vi "Config HW Extract.vi"(4 "Get(f) Set(t)":bool, 6 "Send Cmd Timout(ms)":u32=300, 7 "Drive Refs":T1={"DeviceStatus"={"status"=FALSE, "code"=0, "source"=""}, "Type"=enum."PWM", "PWM"={"PWM Channel"=enum."Invalid", "DeadBand"={"Name"="", "maxPositivePwm"=0, "minPositivePwm"=0, "centerPwm"=0, "maxNegativePwm"=0, "minNegativePwm"=0, "angularRange"=0}}, "CAN"={"Device Number"=0, "SetOutput VI Ref"=variant, "GetOutput VI Ref"=variant, "Enable VI Ref"=variant, "Disable VI Ref"=variant, "Data"=variant}, "Invert"=FALSE, "DIO PWM"={"PWM \"Enable\" Channel"=enum."Invalid", "DIOChannel"=enum."Invalid", "PWM Rate"=0.0}}, 8 "Error":errorcluster, 9 "HW Config":T6={"Drive"={"Drive HW Ver"=0, "SparkMax Output"={"Motor Invert"=FALSE, "Ramp Rate OL (S)"=1.0, "Dead Band"=0.0, "Idle Mode"=enum."Brake"}, "Slot 0 CL"={"Gains"={"P"=0.1, "I"=0.0, "D"=0.0, "F"=0.0}, "I Zone"=0.0, "Peak Out -1 0 1"={"High"=0.0, "Low"=0.0}, "Max I Accu"=0.0}, "Slot 0 SM"={"Max Velocity"=0.0, "Max Acceleration"=0.0, "Allowed CL Error"=0.0, "Min Velocity Output"=0.0}}, "Steer"={"Steer HW Ver"=0, "SRX Output"={"Neutral"=enum."Override to Coast", "Max"={"FWD"=1.0, "REV"=-1.0}, "Min"={"FWD"=1.0, "REV"=-1.0}, "OL Ramp Rate (S)"=0.0, "Dead Band"=0.0, "CL Ramp Rate (S)"=0.0}, "Slot 0 CL"={"Gains"={"P"=1.0, "I"=0.01, "D"=0.0, "F"=0.0}, "Error Allowed"=0.0, "I Zone"=10000.0, "Peak Out 0-1"=1.0, "Max I Accu"=-1000.0}, "Slot 0 MM"={"Cruise Velocity"=5000, "Acceleration"=5000}}} {"Steer"."Slot 0 CL"."Gains"."F" format="%#.8f"; "Steer"."Slot 0 CL"."Gains"."D" format="%#.8f"; "Steer"."Slot 0 CL"."Gains"."I" format="%#.8f"; "Steer"."Slot 0 CL"."Gains"."P" format="%#.8f"; "Steer"."SRX Output"."Min"."REV" format="%.2f"; "Steer"."SRX Output"."Min"."FWD" format="%.2f"; "Steer"."SRX Output"."Max"."REV" format="%.2f"; "Steer"."SRX Output"."Max"."FWD" format="%.2f"; "Drive"."Slot 0 CL"."Gains"."F" format="%#.8f"; "Drive"."Slot 0 CL"."Gains"."D" format="%#.8f"; "Drive"."Slot 0 CL"."Gains"."I" format="%#.8f"; "Drive"."Slot 0 CL"."Gains"."P" format="%#.8f"; "Drive"."Slot 0 CL"."Peak Out -1 0 1"."Low" format="%#.8f"; "Drive"."Slot 0 CL"."Peak Out -1 0 1"."High" format="%#.8f"}, 11 "Steer Refs":T1={"DeviceStatus"={"status"=FALSE, "code"=0, "source"=""}, "Type"=enum."PWM", "PWM"={"PWM Channel"=enum."Invalid", "DeadBand"={"Name"="", "maxPositivePwm"=0, "minPositivePwm"=0, "centerPwm"=0, "maxNegativePwm"=0, "minNegativePwm"=0, "angularRange"=0}}, "CAN"={"Device Number"=0, "SetOutput VI Ref"=variant, "GetOutput VI Ref"=variant, "Enable VI Ref"=variant, "Disable VI Ref"=variant, "Data"=variant}, "Invert"=FALSE, "DIO PWM"={"PWM \"Enable\" Channel"=enum."Invalid", "DIOChannel"=enum."Invalid", "PWM Rate"=0.0}}) -> (0 "Error Out":errorcluster, 1 "HW Config Out":T6={"Drive"={"Drive HW Ver"=0, "SparkMax Output"={"Motor Invert"=FALSE, "Ramp Rate OL (S)"=1.0, "Dead Band"=0.0, "Idle Mode"=enum."Brake"}, "Slot 0 CL"={"Gains"={"P"=0.1, "I"=0.0, "D"=0.0, "F"=0.0}, "I Zone"=0.0, "Peak Out -1 0 1"={"High"=0.0, "Low"=0.0}, "Max I Accu"=0.0}, "Slot 0 SM"={"Max Velocity"=0.0, "Max Acceleration"=0.0, "Allowed CL Error"=0.0, "Min Velocity Output"=0.0}}, "Steer"={"Steer HW Ver"=0, "SRX Output"={"Neutral"=enum."Override to Coast", "Max"={"FWD"=1.0, "REV"=-1.0}, "Min"={"FWD"=1.0, "REV"=-1.0}, "OL Ramp Rate (S)"=0.0, "Dead Band"=0.0, "CL Ramp Rate (S)"=0.0}, "Slot 0 CL"={"Gains"={"P"=1.0, "I"=0.01, "D"=0.0, "F"=0.0}, "Error Allowed"=0.0, "I Zone"=10000.0, "Peak Out 0-1"=1.0, "Max I Accu"=-1000.0}, "Slot 0 MM"={"Cruise Velocity"=5000, "Acceleration"=5000}}} {"Steer"."Slot 0 CL"."Gains"."F" format="%#.8f"; "Steer"."Slot 0 CL"."Gains"."D" format="%#.8f"; "Steer"."Slot 0 CL"."Gains"."I" format="%#.8f"; "Steer"."Slot 0 CL"."Gains"."P" format="%#.8f"; "Steer"."SRX Output"."Min"."REV" format="%.2f"; "Steer"."SRX Output"."Min"."FWD" format="%.2f"; "Steer"."SRX Output"."Max"."REV" format="%.2f"; "Steer"."SRX Output"."Max"."FWD" format="%.2f"; "Drive"."Slot 0 CL"."Gains"."F" format="%#.8f"; "Drive"."Slot 0 CL"."Gains"."D" format="%#.8f"; "Drive"."Slot 0 CL"."Gains"."I" format="%#.8f"; "Drive"."Slot 0 CL"."Gains"."P" format="%#.8f"; "Drive"."Slot 0 CL"."Peak Out -1 0 1"."Low" format="%#.8f"; "Drive"."Slot 0 CL"."Peak Out -1 0 1"."High" format="%#.8f"}, 3 "Steer Refs Out":T1={"DeviceStatus"={"status"=FALSE, "code"=0, "source"=""}, "Type"=enum."PWM", "PWM"={"PWM Channel"=enum."Invalid", "DeadBand"={"Name"="", "maxPositivePwm"=0, "minPositivePwm"=0, "centerPwm"=0, "maxNegativePwm"=0, "minNegativePwm"=0, "angularRange"=0}}, "CAN"={"Device Number"=0, "SetOutput VI Ref"=variant, "GetOutput VI Ref"=variant, "Enable VI Ref"=variant, "Disable VI Ref"=variant, "Data"=variant}, "Invert"=FALSE, "DIO PWM"={"PWM \"Enable\" Channel"=enum."Invalid", "DIOChannel"=enum."Invalid", "PWM Rate"=0.0}}, 5 "Drive Refs Out":T1={"DeviceStatus"={"status"=FALSE, "code"=0, "source"=""}, "Type"=enum."PWM", "PWM"={"PWM Channel"=enum."Invalid", "DeadBand"={"Name"="", "maxPositivePwm"=0, "minPositivePwm"=0, "centerPwm"=0, "maxNegativePwm"=0, "minNegativePwm"=0, "angularRange"=0}}, "CAN"={"Device Number"=0, "SetOutput VI Ref"=variant, "GetOutput VI Ref"=variant, "Enable VI Ref"=variant, "Disable VI Ref"=variant, "Data"=variant}, "Invert"=FALSE, "DIO PWM"={"PWM \"Enable\" Channel"=enum."Invalid", "DIOChannel"=enum."Invalid", "PWM Rate"=0.0}})   [LabVIEW 2023, in "Swerve AM_ACT.lvlib"]
uses:
  Swerve AM_ACT.lvlib
  Shared Code/TypeDefs/Cluster_PID Gains.ctl
  Shared Code/TypeDefs/Cluster_SRX SLOT PID Config.ctl
  <vilib>/Rock Robotics/WPI/ThirdParty/Phoenix-LabVIEW/Motor Controller/Controls/CTRE_Phoenix_MotorControl_NeutralMode.ctl
  Shared Code/TypeDefs/Cluster_FWD  REV Values.ctl
  Shared Code/TypeDefs/Cluster_Config SRX Motor Output.ctl
  Cluster_Config HW Values.ctl
  Cluster_Config Drive HW Values.ctl
  Cluster_Config Steer HW Values.ctl
  <vilib>/Rock Robotics/SystemInterfaces/DIO/FPGA_DIOPWMChannel.ctl
  <vilib>/Rock Robotics/WPI/PWM/WPI_PWMDeadband.ctl
  <vilib>/Rock Robotics/WPI/MotorControl/WPI_MotorControlType.ctl
  <vilib>/Rock Robotics/SystemInterfaces/DIO/FPGA_DIOChannel.ctl
  <vilib>/Rock Robotics/WPI/MotorControl/WPI_MotorControlDeviceRef.ctl
  <vilib>/Rock Robotics/WPI/ThirdParty/REV Robotics/REVLib/Typedef/Spark MAX Idle Mode.ctl
  Shared Code/TypeDefs/Cluster_High-Low.ctl
  Shared Code/TypeDefs/Cluster_Spark MAX Config_SLOT PID Config.ctl
  Shared Code/TypeDefs/Cluster_SparkMax Config_Motor Output.ctl
  Shared Code/TypeDefs/Cluster_SparkMax Config_Smart Motion Parameters.ctl
  Shared Code/TypeDefs/Cluster_SRX Motion Magic Parameters.ctl
panel:
  # "Tune Output\nto 1023 Max"
  # "Tune Output\nto 1023 Max"
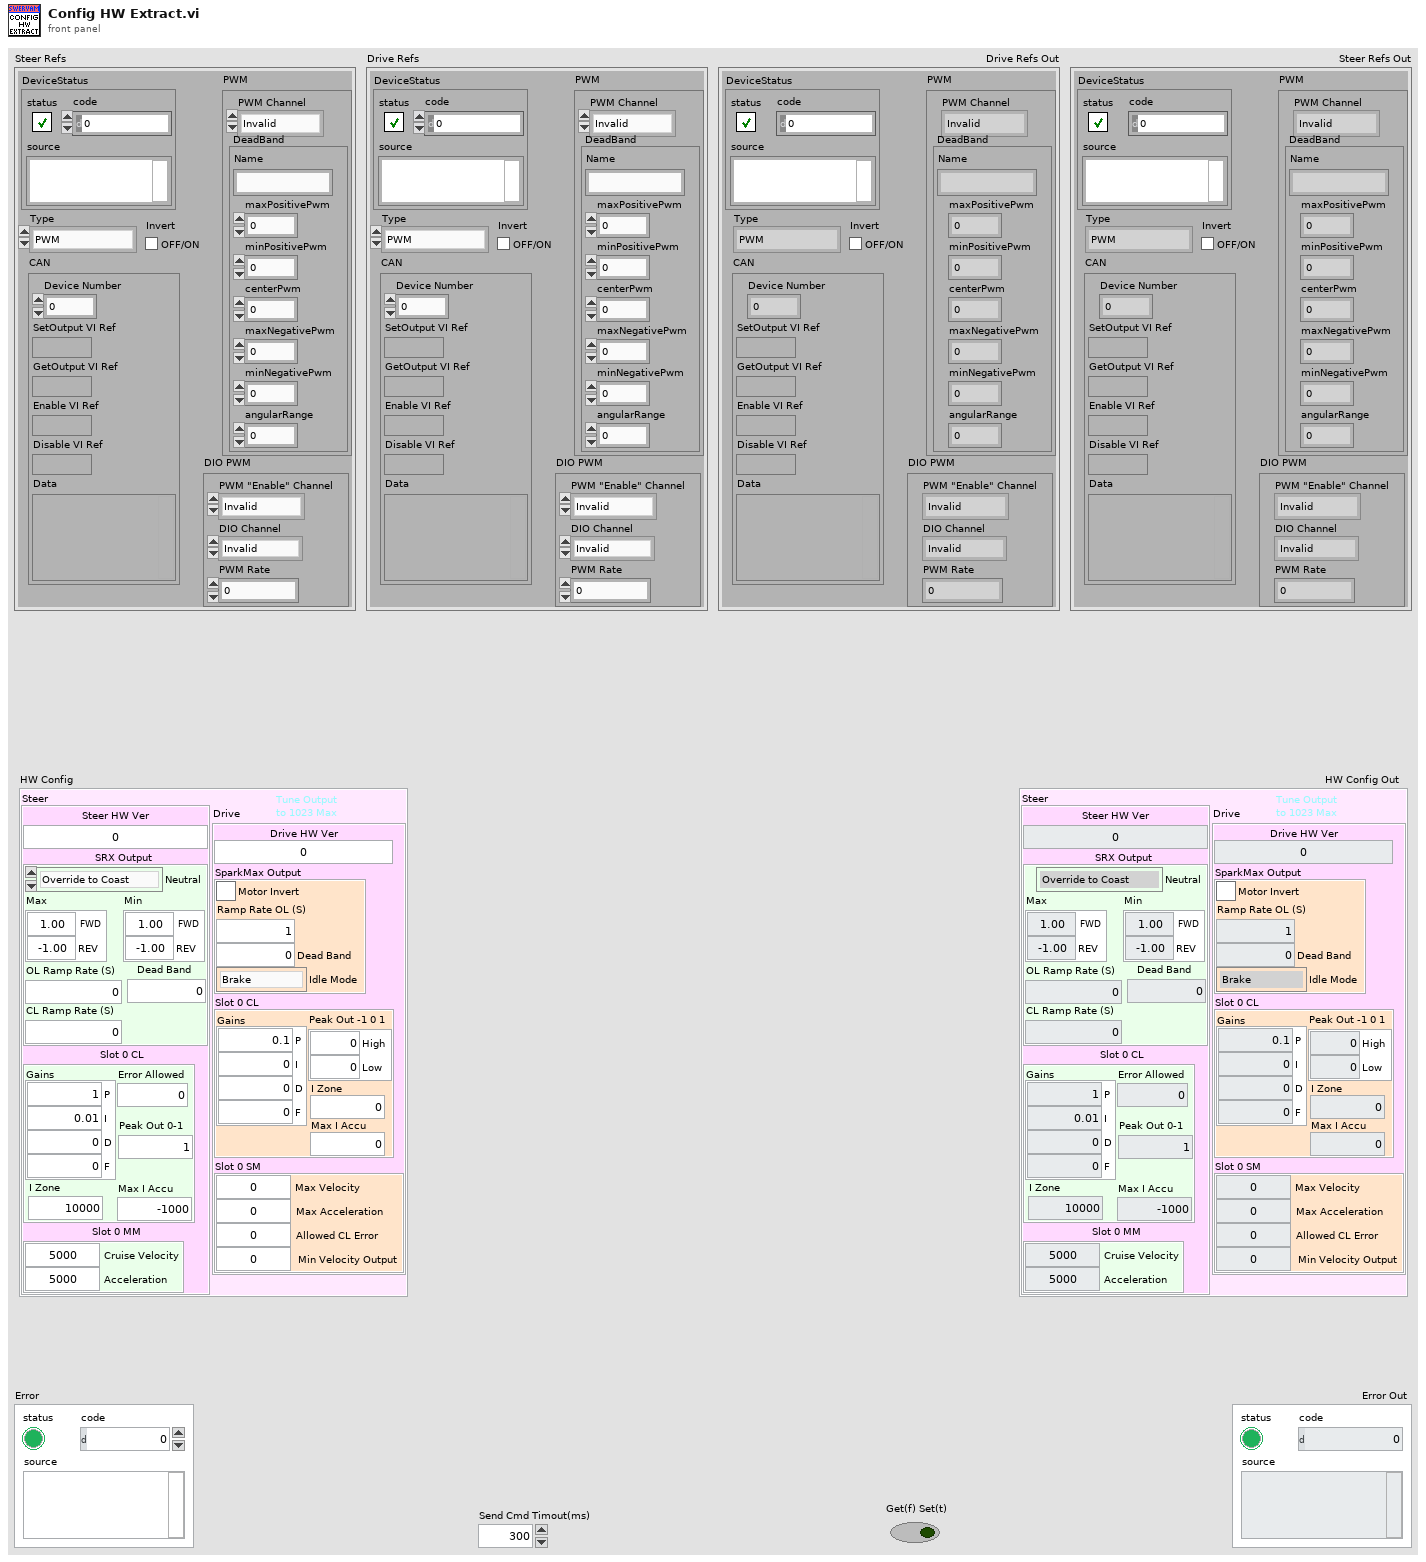
[diagram p1: front panel]
types:
  T1 = typedef "WPI_MotorControlDeviceRef.ctl" = cluster{"DeviceStatus":errorcluster, "Type":T2, "PWM":cluster{"PWM Channel":T3, "DeadBand":T4}, "CAN":cluster{"Device Number":u8, "SetOutput VI Ref":variant, "GetOutput VI Ref":variant, "Enable VI Ref":variant, "Disable VI Ref":variant, "Data":variant}, "Invert":bool, "DIO PWM":cluster{"PWM \"Enable\" Channel":T3, "DIOChannel":T5, "PWM Rate":dbl}}
  T2 = typedef "WPI_MotorControlType.ctl" = enum16{"PWM", "CAN", "DIO PWM"}
  T3 = typedef "FPGA_DIOPWMChannel.ctl" = enum8{"PWM 0", "PWM 1", "PWM 2", "PWM 3", "PWM 4", "PWM 5", "PWM 6", "PWM 7", "PWM 8", "PWM 9", "PWM MXP 0", "PWM MXP 1", "PWM MXP 2", "PWM MXP 3", "PWM MXP 4", "PWM MXP 5", "PWM MXP 6", "PWM MXP 7", "PWM MXP 8", "PWM MXP 9", "Invalid"}
  T4 = typedef "WPI_PWMDeadband.ctl" = cluster{"Name":string, "maxPositivePwm":i32, "minPositivePwm":i32, "centerPwm":i32, "maxNegativePwm":i32, "minNegativePwm":i32, "angularRange":u16}
  T5 = typedef "FPGA_DIOChannel.ctl" = enum8{"DIO 0", "DIO 1", "DIO 2", "DIO 3", "DIO 4", "DIO 5", "DIO 6", "DIO 7", "DIO 8", "DIO 9", "DIO MXP 0", "DIO MXP 1", "DIO MXP 2", "DIO MXP 3", "DIO MXP 4", "DIO MXP 5", "DIO MXP 6", "DIO MXP 7", "DIO MXP 8", "DIO MXP 9", "DIO MXP 10", "DIO MXP 11", "DIO MXP 12", "DIO MXP 13", "DIO MXP 14", "DIO MXP 15", "SPI Port CS1", "SPI Port CS2", "SPI Port CS3", "SPI Port MISO", "SPI Port MOSI", "Invalid"}
  T6 = typedef "Swerve AM_ACT.lvlib/Cluster_Config HW Values.ctl" = cluster{"Drive":T7, "Steer":T14}
  T7 = typedef "Swerve AM_ACT.lvlib/Cluster_Config Drive HW Values.ctl" = cluster{"Drive HW Ver":u64, "SparkMax Output":T8, "Slot 0 CL":T10, "Slot 0 SM":T13}
  T8 = typedef "Cluster_SparkMax Config_Motor Output.ctl" = cluster{"Motor Invert":bool, "Ramp Rate OL (S)":dbl, "Dead Band":dbl, "Idle Mode":T9}
  T9 = typedef "Spark MAX Idle Mode.ctl" = enum16{"Coast", "Brake"}
  T10 = typedef "Cluster_Spark MAX Config_SLOT PID Config.ctl" = cluster{"Gains":T11, "I Zone":dbl, "Peak Out -1 0 1":T12, "Max I Accu":dbl}
  T11 = typedef "Cluster_PID Gains.ctl" = cluster{"P":dbl, "I":dbl, "D":dbl, "F":dbl}
  T12 = typedef "Cluster_High-Low.ctl" = cluster{"High":dbl, "Low":dbl}
  T13 = typedef "Cluster_SparkMax Config_Smart Motion Parameters.ctl" = cluster{"Max Velocity":dbl, "Max Acceleration":dbl, "Allowed CL Error":dbl, "Min Velocity Output":dbl}
  T14 = typedef "Swerve AM_ACT.lvlib/Cluster_Config Steer HW Values.ctl" = cluster{"Steer HW Ver":u64, "SRX Output":T15, "Slot 0 CL":T18, "Slot 0 MM":T19}
  T15 = typedef "Cluster_Config SRX Motor Output.ctl" = cluster{"Neutral":T16, "Max":T17, "Min":T17, "OL Ramp Rate (S)":dbl, "Dead Band":dbl, "CL Ramp Rate (S)":dbl}
  T16 = typedef "CTRE_Phoenix_MotorControl_NeutralMode.ctl" = enum8{"EEPROMSetting", "Override to Coast", "Override to Brake"}
  T17 = typedef "Cluster_FWD  REV Values.ctl" = cluster{"FWD":dbl, "REV":dbl}
  T18 = typedef "Cluster_SRX SLOT PID Config.ctl" = cluster{"Gains":T11, "Error Allowed":dbl, "I Zone":dbl, "Peak Out 0-1":dbl, "Max I Accu":dbl}
  T19 = typedef "Cluster_SRX Motion Magic Parameters.ctl" = cluster{"Cruise Velocity":i32, "Acceleration":i32}
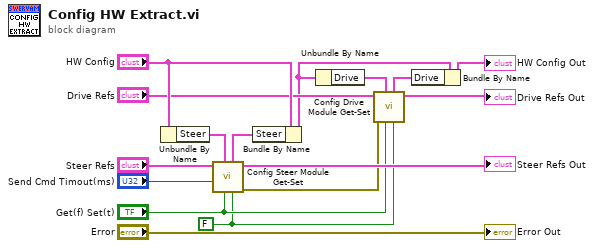
[diagram p0: block diagram]
diagram:
  w1 = FALSE ("Start with Default")
  n1 = Unbundle By Name("HW Config") -> ("Steer"=w7:T14)
  n2 = call "Config Steer Module Get-Set.vi"("Start With Default"=w1, "Get(f) Set(t)"="Get(f) Set(t)", "Set Steer Values"=w7, "Send Cmd Timout(ms)"="Send Cmd Timout(ms)", "Steer Refs"="Steer Refs") -> ("Error Out"=w5:errorcluster, "Steer Refs Out"=→"Steer Refs Out":T1, "Steer Config Out"=w6:T14)  [unwired: 3 in, 1 out]
  n3 = Bundle By Name(cluster="HW Config", "Steer"=w6) -> (w3:T6)
  n4 = Unbundle By Name(w3) -> ("Drive"=w4:T7)
  n5 = call "Config Drive Module Get-Set.vi"("Start with Default"=w1, "Get(f) Set(t)"="Get(f) Set(t)", "Set Drive Config"=w4, "Error"=w5, "Drive Refs"="Drive Refs") -> ("Drive Refs Out"=→"Drive Refs Out":T1, "Drive Config Out"=w2:T7)  [unwired: 4 in, 1 out]
  n6 = Bundle By Name(cluster=w3, "Drive"=w2) -> (→"HW Config Out":T6)
  "Error Out" <- "Error"
